vi "calibrationWriter.vi"() -> ()   [LabVIEW 2014]
uses:
  <vilib>/Utility/file.llb/Write To Spreadsheet File (string).vi
panel:
  in  "Pulse Duration":dbl[](array[numeric])
  in  "Probe #":dbl[](array[numeric])
  in  "0 weight":dbl[](array[numeric])
  in  "Pulses":dbl[][](array[numeric])
  in  "Weight":dbl[][](array[numeric])
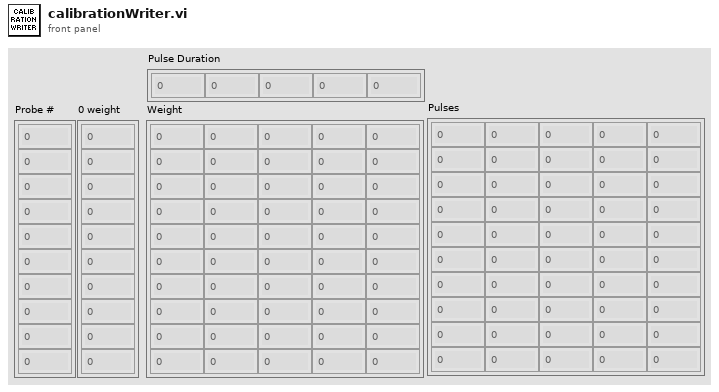
[diagram p1: front panel]
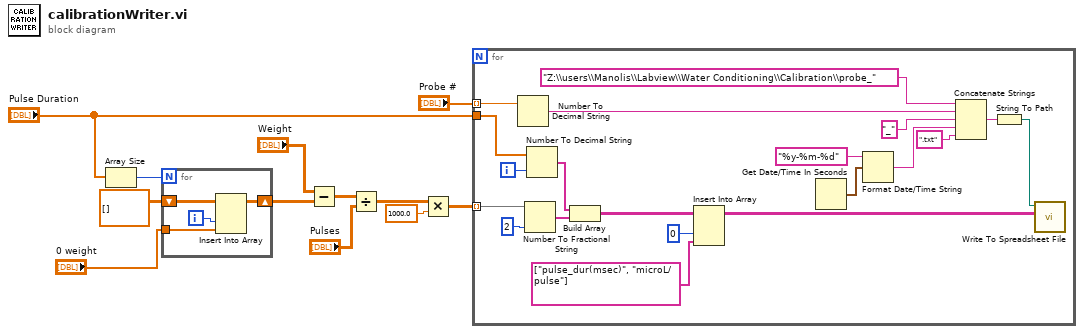
[diagram p0: block diagram]
diagram:
  n1 = Array Size(array="Pulse Duration") -> (size(s)=w11:i32)
  n2 = for {
    N: w11 -> [_]
    shift-right: [w15] -> w9
    shift-left: dbl[][] [] -> [w16]
    tunnel: "0 weight" -> [w13]
    i -> [w14]
    n3 = Insert Into Array(array=w16, index (col)=w14, new element=w13) -> (w15:dbl[][])  [unwired: 1 in]
  }
  n4 = Subtract(x="Weight", y=w9) -> (x-y=w7:dbl[][])
  n5 = Divide(x=w7, y="Pulses") -> (x/y=w2:dbl[][])
  n6 = Multiply(x=w2, y=1000.0) -> (x*y=w1:dbl[][])
  n7 = for {
    tunnel: w1 -> [w20] mode=indexing
    tunnel: "Pulse Duration" -> [w22]
    tunnel: "Probe #" -> [w35] mode=indexing
    i -> [w23]
    n8 = Number To Decimal String(number=w35) -> (decimal integer string=w34:string)  [unwired: 1 in]
    n9 = Number To Fractional String(number=w20, precision (6)=i16 2) -> (F-format string=w18:string[])  [unwired: 2 in]
    n10 = Number To Decimal String(number=w22, width (-)=w23) -> (decimal integer string=w21:string[])
    n11 = Build Array(w21, w18) -> (w17:string[][])
    n12 = Insert Into Array(array=w17, index (col)=0 ("disabled index (col)"), new element=string[] ["pulse_dur(msec)", "microL/pulse"]) -> (w24:string[][])  [unwired: 1 in]
    n13 = Get Date/Time In Seconds() -> (seconds since 1Jan1904=w32:timestamp)
    n14 = Format Date/Time String(time format string (%c)="%y-%m-%d", seconds (now)=w32) -> (date/time string=w29:string)  [unwired: 1 in]
    n15 = Concatenate Strings("Z:\\users\\Manolis\\Labview\\Water Conditioning\\Calibration\\probe_", w34, "_" ("string"), w29, ".txt" ("string")) -> (w28:string)
    n16 = String To Path(string=w28) -> (path=w27:path)
    n17 = call-poly <vilib>:"Write To Spreadsheet File.vi"("2D data"=w24, "file path (dialog if empty)"=w27) -> ()  [unwired: 6 in, 1 out]
  }
